vi "set endianness.vi"(8 "error in":errorcluster, 10 "byte orders":T6[](array[typedef]), 11 "config in":T1[](array[typedef])) -> (0 "error out":errorcluster, 3 "config out":T1[](array[typedef]))   [LabVIEW 2013, in "Profibus Module runtime.lvclass"]
uses:
  Profibus Module runtime.lvclass
  configuration/endianness setting.ctl
  profibus slave configuration.ctl
  profibus mapping configuration.ctl
  <vilib>/NI/Tag Bus/tag/Data Type.ctl
  dynamic profibus/full command.ctl
  dynamic profibus/profibus master action.ctl
  configuration/Profibus Module configuration.lvclass
  <vilib>/NI/Tag Bus/tag/tag descriptor.lvclass
  dynamic profibus/dynamic profibus.lvlib
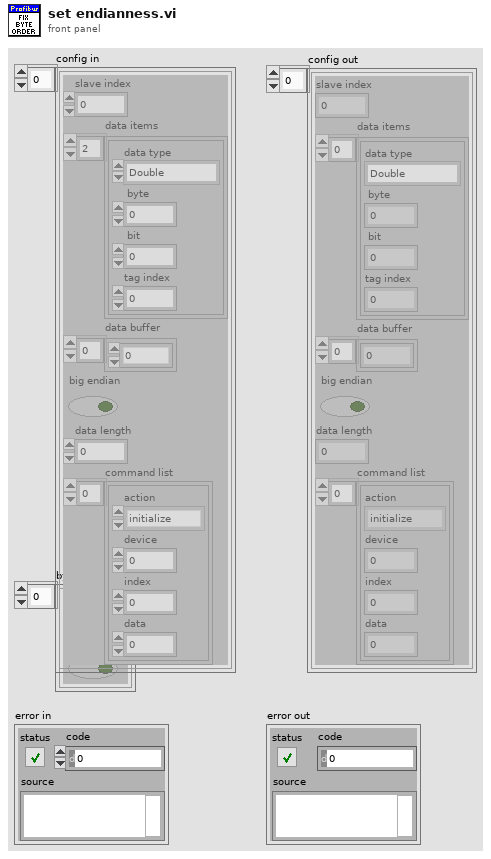
[diagram p1: front panel]
types:
  T1 = typedef "Profibus Module runtime.lvclass/profibus slave configuration.ctl" = cluster{"slave index":i8, "data items":T2[], "data buffer":u8[], "big endian":bool, "data length":i32, "command list":T4[]}
  T2 = typedef "Profibus Module runtime.lvclass/profibus mapping configuration.ctl" = cluster{"data type":T3, " byte":i32, " bit":i32, "tag index":i32}
  T3 = typedef "tag bus.lvlib/tag descriptor.lvclass/Data Type.ctl" = enum16{"Double", "Single", "I64", "I32", "I16", "I8", "U64", "U32", "U16", "U8", "Boolean", "String", "Array of Double", "Array of Single", "Array of I64", "Array of I32", "Array of I16", "Array of I8", "Array of U64", "Array of U32", "Array of U16", "Array of U8", "Array of Boolean", "Array of String"}
  T4 = typedef "dynamic profibus.lvlib/full command.ctl" = cluster{"action":T5, "device":u8, "index":u8, "data":u8}
  T5 = typedef "dynamic profibus.lvlib/profibus master action.ctl" = enum8{"initialize", "uninitialize", "stop", "get input", "get input size", "set output", "get output size", "get diagnostic", "transfer data", "transfer diagnostics"}
  T6 = typedef "Profibus Module configuration.lvclass/endianness setting.ctl" = cluster{"slave":i8, "big endian":bool}
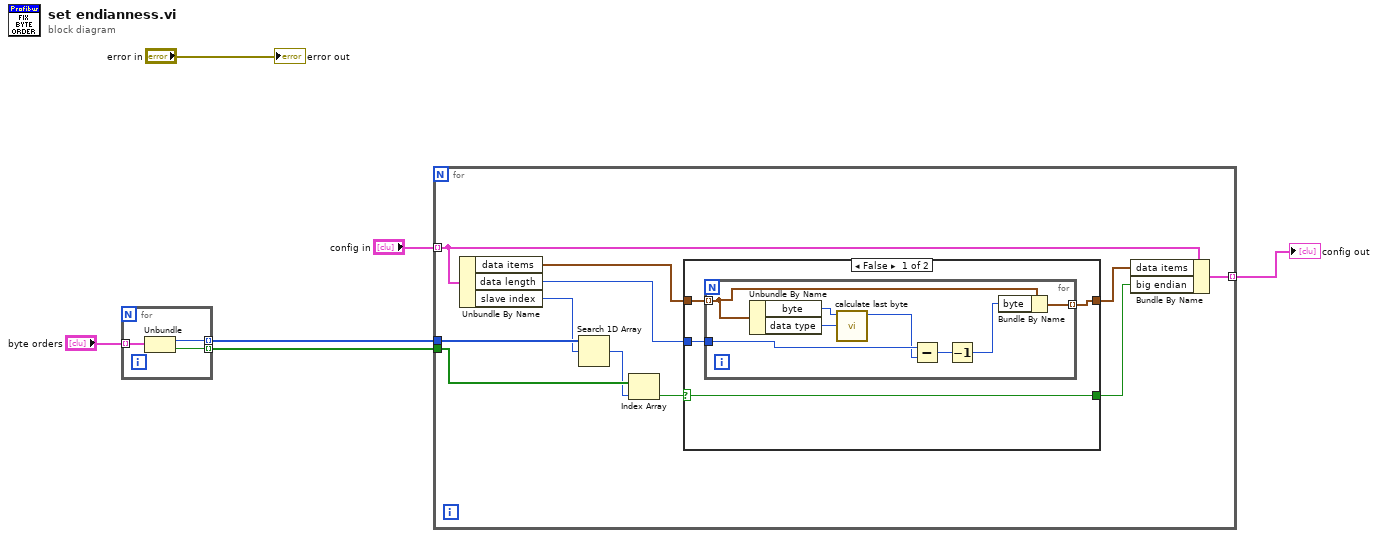
[diagram p0: block diagram]
diagram:
  n1 = for {
    tunnel: "byte orders" -> [w9] mode=indexing
    tunnel: [w8] -> w4 mode=indexing
    tunnel: [w7] -> w3 mode=indexing
    n2 = Unbundle(w9) -> ("slave"=w8:i8, "big endian"=w7:bool)
  }
  n3 = for {
    tunnel: "config in" -> [w16] mode=indexing
    tunnel: w4 -> [w20]
    tunnel: w3 -> [w18]
    tunnel: [w15] -> w2 mode=indexing
    n4 = Unbundle By Name(w16) -> ("data items"=w11:T2[], "data length"=w10:i32, "slave index"=w19:i8)
    n5 = Search 1D Array(1D array=w20, element=w19) -> (index of element=w17:i32)  [unwired: 1 in]
    n6 = Index Array(array=w18, index=w17) -> (element=w14:bool)
    n7 = case shown="False" w14 {
      selector: w14 -> [w24 w34]
      tunnel: [w24 w34] -> w13
      tunnel: [w21 w33] -> w12
      tunnel: w11 -> [w23 w33]
      tunnel: w10 -> [w22 _]
      frame False {
        n8 = for {
          tunnel: w23 -> [w30] mode=indexing
          tunnel: w22 -> [w28]
          tunnel: [w29] -> w21 mode=indexing
          n9 = Unbundle By Name(w30) -> ("byte"=w32:i32, "data type"=w31:T3)
          n10 = call "calculate last byte.vi"("type"=w31, "byte in"=w32) -> ("last byte"=w27:i32)  [unwired: 9 in]
          n11 = Subtract(x=w28, y=w27) -> (x-y=w26:i32)
          n12 = Decrement(x=w26) -> (x-1=w25:i32)
          n13 = Bundle By Name(cluster=w30, "byte"=w25) -> (w29:T2)
        }
      }
      frame True {
      }
    }
    n14 = Bundle By Name(cluster=w16, "data items"=w12, "big endian"=w13) -> (w15:T1)
  }
  "config out" <- w2
  "error out" <- "error in"
